vi "set ParentNode.vi"(8 "error in (no error)":errorcluster caption="错误输入（无错误）", 10 "ParentNode*":refnum<data-value>, 11 "PanelLinkNode输入":refnum<class "PanelLinkNode.lvclass">) -> (0 "error out":errorcluster caption="错误输出", 3 "PanelLinkNode输出":refnum<class "PanelLinkNode.lvclass">)   [LabVIEW 2013, in "PanelLinkNode.lvclass"]
uses:
  PanelLinkNode.lvclass
  PanelObject/PanelObject.lvclass
  PanelLinkNode.lvclass/PanelLinkNode.ctl
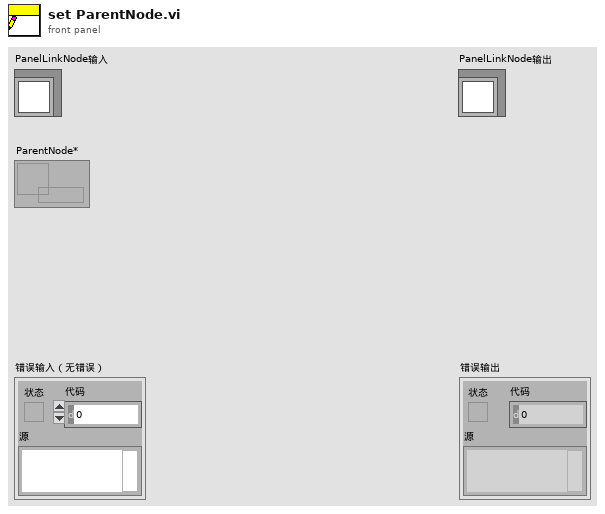
[diagram p1: front panel]
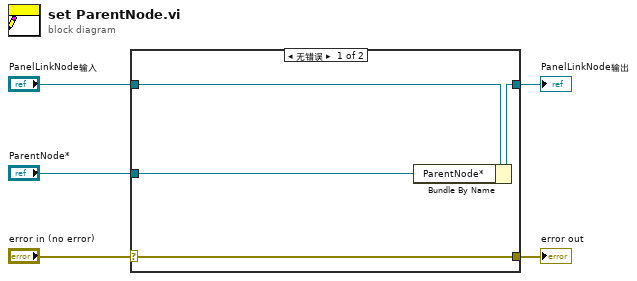
[diagram p0: block diagram]
diagram:
  n1 = case shown="无错误" "error in (no error)" {
    selector: "error in (no error)" -> [w9 w10]
    tunnel: [w9 w10] -> w4
    tunnel: [w7 w11] -> w2
    tunnel: "PanelLinkNode输入" -> [w8 w11]
    tunnel: "ParentNode*" -> [w6 _]
    frame No Error {
      n2 = Bundle By Name(cluster=w8, "ParentNode*"=w6) -> (w7:refnum<class "PanelLinkNode.lvclass">)
    }
    frame Error {
    }
  }
  "error out" <- w4
  "PanelLinkNode输出" <- w2
